vi "SSL_Query.vi"(0 "System no.":i32=1 min=1 max=4 step=1, 2 "Axes to query":string[](array[string]), 3 "All axes?":bool, 4 "Axis identifier?":bool=TRUE, 5 "error in":errorcluster) -> (14 "Softlimit status?":bool[](array[boolean]), 19 "error out":errorcluster)   [LabVIEW 2020]
doc: "Returns soft-limit status for queried axes.\n\nC-702: If All axes = TRUE, then Axis identifier can be FALSE\nC-844: If All axes = TRUE, then Axis identifier can be FALSE\nC-848: If All axes = TRUE, then Axis identifier can be FALSE\nC-880: If All axes = TRUE, then Axis identifier can be FALSE\nC-886: If All axes = TRUE, then Axis identifier can be FALSE\nE-755: If All axes? = TRUE, then Axis identifier? can be FALSE. Command not available for E-755.101.\nC-887, F-206, M-8X0: If All axes? = TRUE, then Axis identifier? can be FALSE."
panel:
  # "Returns softlimit status for queried axes."
  # "If all axes: use"
  # "Query"
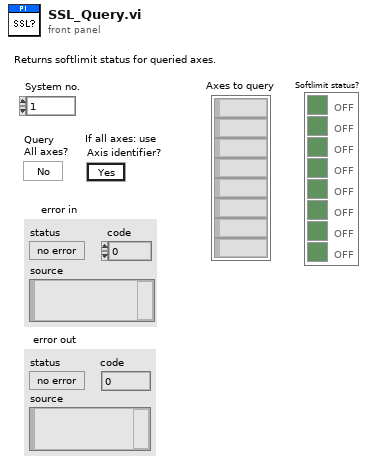
[diagram p1: front panel]
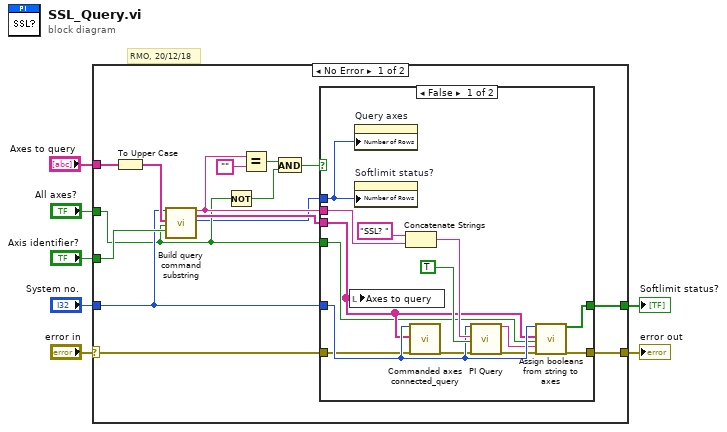
[diagram p0: block diagram]
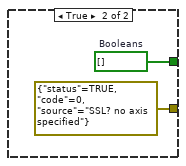
[diagram p2: hidden frame]
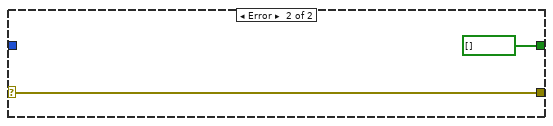
[diagram p3: hidden frame]
diagram:
  # "RMO, 20/12/18"
  n1 = case shown="No Error" "error in" {
    selector: "error in" -> [w10 w39]
    tunnel: [w22 bool[] [] ("Booleans")] -> w7
    tunnel: "Axes to query" -> [w21 _]
    tunnel: [w9 w39] -> w5
    tunnel: "Axis identifier?" -> [w18 _]
    tunnel: "System no." -> [w16 _]
    tunnel: "All axes?" -> [w14 _]
    frame No Error {
      n2 = To Upper Case(1:w21) -> (0:w19:string[])
      n3 = call "Build query command substring.vi"("System no."=w16, "Axes to query in"=w19, "Query\nAll axes?"=w14, "For all axes: use\nAxis identifier?"=w18) -> ("Command substring"=w17:string, "Axes to query out"=w15:string[], "Number of rows"=w11:u32)  [unwired: 2 in, 11 out]
      n4 = Not(x=w14) -> (.not. x?=w12:bool)
      n5 = Equal?(x=w17, y="" ("x")) -> (x = y?=w13:bool)
      n6 = And(x=w13, y=w12) -> (x .and. y?=w8:bool)
      n7 = case shown="False" w8 {
        tunnel: [w33 w37] -> w22
        tunnel: w17 -> [w32 _]
        tunnel: w16 -> [w31 _]
        tunnel: w15 -> [w30 _]
        tunnel: w14 -> [w29 _]
        tunnel: w11 -> [w28 _]
        tunnel: w10 -> [w26 _]
        tunnel: [w25 errorcluster {"status"=TRUE, "code"=0, "source"="SSL? no axis specified"} ("error out")] -> w9
        frame False {
          n8 = local write "Axes to query"(w30) -> ()
          n9 = property on="Query axes" class="Arr (strict)"("Number of Rows"=w28) -> ()  [unwired: 2 in, 2 out]
          n10 = property on="Softlimit status?" class="Arr (strict)"("Number of Rows"=w28) -> ()  [unwired: 2 in, 2 out]
          n11 = Concatenate Strings("SSL? ", w32) -> (w34:string)
          n12 = call "Commanded axes connected_query.vi"("System no."=w31, "Commanded axes"=w30, "error in"=w26) -> ("error out"=w27:errorcluster)  [unwired: 1 in, 15 out]
          n13 = call "PI Query.vi"("System no."=w31, "String to send"=w34, "Attach termination char.?"=TRUE ("Attach Linefeed?"), "error in"=w27) -> ("String read"=w23:string, "error out"=w24:errorcluster)  [unwired: 3 in, 11 out]
          n14 = call "Assign booleans from string to axes.vi"("System no."=w31, "Queried axes"=w30, "All axes queried?"=w29, "Input String"=w23, "error in"=w24) -> ("Booleans"=w33:bool[], "error out"=w25:errorcluster)  [unwired: 13 out]
        }
        frame True {
          w37 = bool[] []  # Booleans
        }
      }
    }
    frame Error {
    }
  }
  "error out" <- w5
  "Softlimit status?" <- w7
